vi "Prepare for Discovery from Loaders.vi"(8 "error in (no error)":errorcluster, 10 "Update Metadata":bool, 11 "CIFPluginManager in":refnum<class "CIFPluginManager.lvclass">) -> (0 "error out":errorcluster)   [LabVIEW 2021, in "CIFPluginManager.lvclass"]
uses:
  CIFPluginManager.lvclass
  typedef/Loader Type.ctl
  CIFPluginManager.lvclass/CIFPluginManager.ctl
  typedef/Loader Load Command.ctl
  typedef/Discover Command.ctl
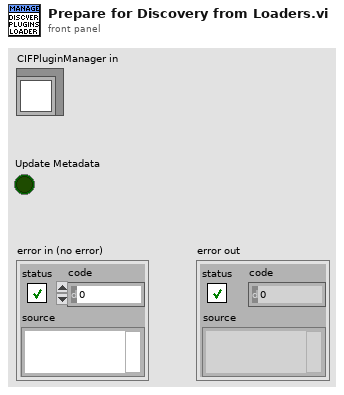
[diagram p1: front panel]
types:
  T1 = typedef "CIFPluginManager.lvclass/Loader Type.ctl" = enum16{"LabVIEW"}
  T2 = typedef "CIFPluginManager.lvclass/Loader Map.ctl" = map{string, T3}
  T3 = typedef "CIFPluginManager.lvclass/Loaders.ctl" = cluster{"Loader Type":T1, "grpc_port":i32, "pid":u32, "gRPC ID":T4, "Load Timestamp":i64, "Unloading":bool, "Ready for removal":bool, "Unload Timestamp":i64}
  T4 = typedef "grpc-lvsupport-release.lvlib/grpcId.ctl" = u64
  T5 = typedef "CIFPluginManager.lvclass/Discover Command.ctl" = cluster{"Loader Name":string, "Update Metadata":bool}
  T6 = typedef "CIFPluginManager.lvclass/Loader Load Command.ctl" = cluster{"Loader Type":T1, "Loader Name":string}
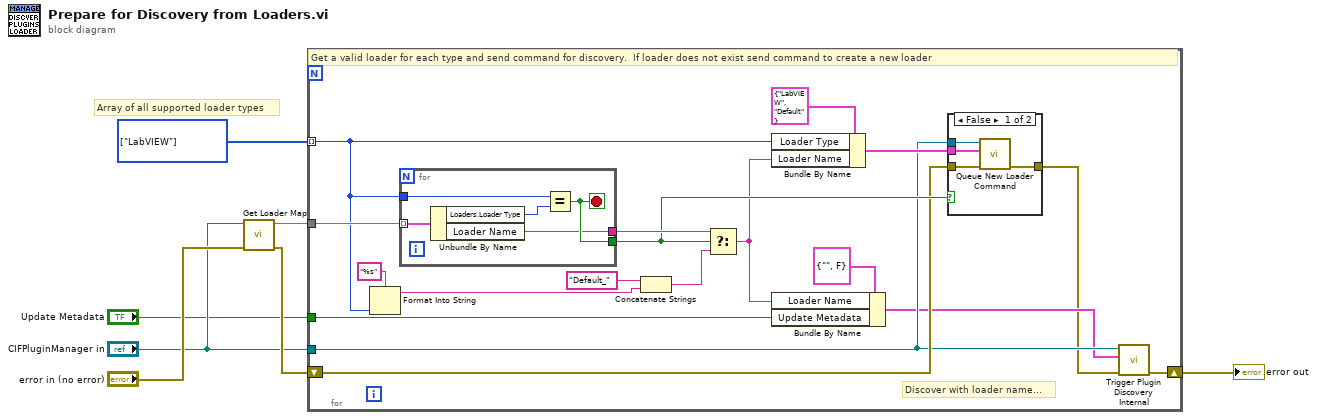
[diagram p0: block diagram]
diagram:
  w1 = T1[] [enum."LabVIEW"] items=["LabVIEW"]
  # "Array of all supported loader types"
  n1 = call "Get Loader Map.vi"("error in (no error)"="error in (no error)", "CIFPluginManager in"="CIFPluginManager in") -> ("error out"=w5:errorcluster, "Loader Map"=w7:T2)  [unwired: 8 in]
  n2 = for {
    tunnel: w7 -> [w25]
    tunnel: "CIFPluginManager in" -> [w19]
    tunnel: "Update Metadata" -> [w16]
    shift-right: [w13] -> w2
    shift-left: w5 -> [w20]
    tunnel: w1 -> [w10] mode=indexing
    # "Discover with loader name..."
    # "Get a valid loader for each type and send command for discovery.  If loader does not exist send command to create a new loader"
    n3 = Format Into String(format string="%s", w10) -> (resulting string=w8:string)  [unwired: 2 in, 1 out]
    n4 = for {
      tunnel: w25 -> [w35] mode=indexing
      tunnel: w10 -> [w34]
      tunnel: [w33] -> w23
      tunnel: [w32] -> w24
      stop <- w33 stop-if-true
      n5 = Unbundle By Name(w35) -> ("Loaders.Loader Type"=w31:T1, "Loader Name"=w32:string)
      n6 = Equal?(x=w34, y=w31) -> (x = y?=w33:bool)
    }
    n7 = Concatenate Strings("Default_" ("f"), w8) -> (w11:string)
    n8 = Select(t=w24, s=w23, f=w11) -> (s? t:f=w17:string)
    n9 = Bundle By Name(cluster=T6 {"Loader Type"=enum."LabVIEW", "Loader Name"="Default"} ("New Launcher"), "Loader Type"=w10, "Loader Name"=w17) -> (w21:T6)
    n10 = Bundle By Name(cluster=T5 {"Loader Name"="", "Update Metadata"=FALSE} ("Trigger Discovery"), "Loader Name"=w17, "Update Metadata"=w16) -> (w15:T5)
    n11 = case shown="False" w23 {
      tunnel: w21 -> [w29 _]
      tunnel: w19 -> [w28 _]
      tunnel: w20 -> [w27 w30]
      tunnel: [w26 w30] -> w14
      frame False {
        n12 = call "Queue New Loader Command.vi"("error in (no error)"=w27, "New Launcher"=w29, "CIFPluginManager in"=w28) -> ("error out"=w26:errorcluster)  [unwired: 8 in]
      }
      frame True {
      }
    }
    n13 = call "Trigger Plugin Discovery Internal.vi"("error in (no error)"=w14, "Trigger Discovery"=w15, "CIFPluginManager in"=w19) -> ("error out"=w13:errorcluster)  [unwired: 8 in]
  }
  "error out" <- w2
